vi "miopen.vi"(2 "错误输入（无错误）":errorcluster, 3 "name":string, 4 "port":u16=1234, 5 "ip":string="127.0.0.1") -> (0 "错误输出":errorcluster, 1 "连接ID":refnum<k5>)   [LabVIEW 2017]
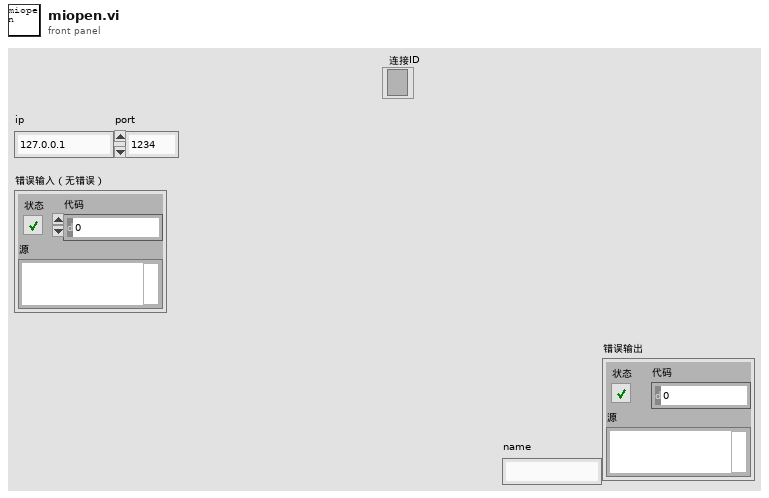
[diagram p1: front panel]
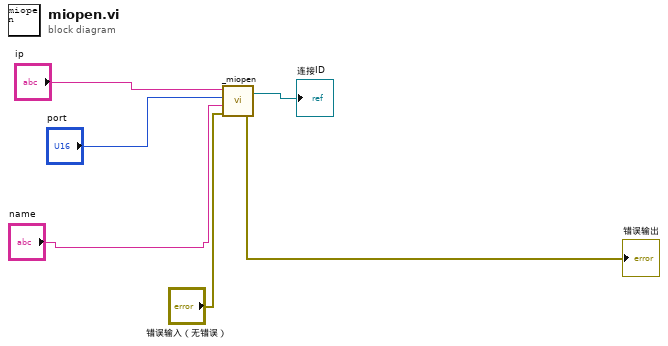
[diagram p0: block diagram]
diagram:
  n1 = call "_miopen.vi"("错误输入（无错误）"="错误输入（无错误）", "数据输入"="name", "port"="port", "ip"="ip") -> ("错误输出"=→"错误输出":errorcluster, "连接ID"=→"连接ID":refnum<k5>)
